vi "G#SubTemplateG3_Create.vi"(0 "reference in":refnum<class "G#SubTemplateG3.lvclass">, 5 "error in (no error)":errorcluster) -> (14 "reference out":refnum<class "G#SubTemplateG3.lvclass">, 19 "error out":errorcluster)   [LabVIEW 2020, in "G#SubTemplateG3.lvclass"]
doc: "Constructor."
uses:
  G#SubTemplateG3.lvclass
  C:/ProjectGSharpDevelopment_2020-3/gsharp/VIPM/Files/vi.lib/addons/_AddQ/G#Object/G#Object.lvclass
  C:/ProjectGSharpDevelopment_2020-3/gsharp/VIPM/Files/vi.lib/addons/_AddQ/G#Templates/G#BaseTemplateG3/G#BaseTemplateG3.lvclass
  G#Object/G#Object.lvclass
  G#BaseTemplateG3/G#BaseTemplateG3.lvclass
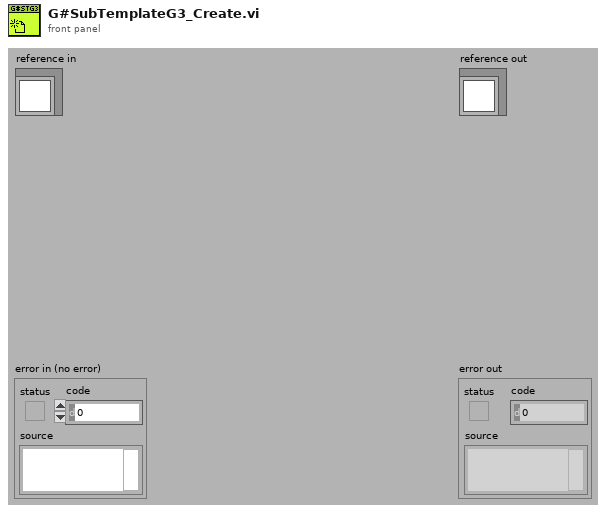
[diagram p1: front panel]
types:
  T1 = typedef "G#SubTemplateG3.lvclass/ObjectAttributes.ctl" = cluster{"Base class":T2}
  T2 = typedef "G#BaseTemplateG3.lvclass/ObjectAttributes.ctl" = cluster{"Numeric":dbl, "String":string, "Boolean":bool}
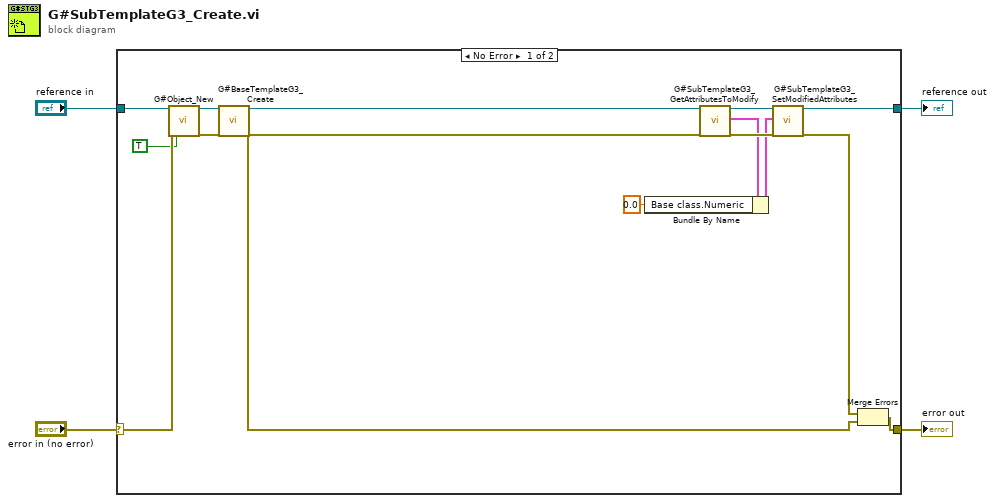
[diagram p0: block diagram]
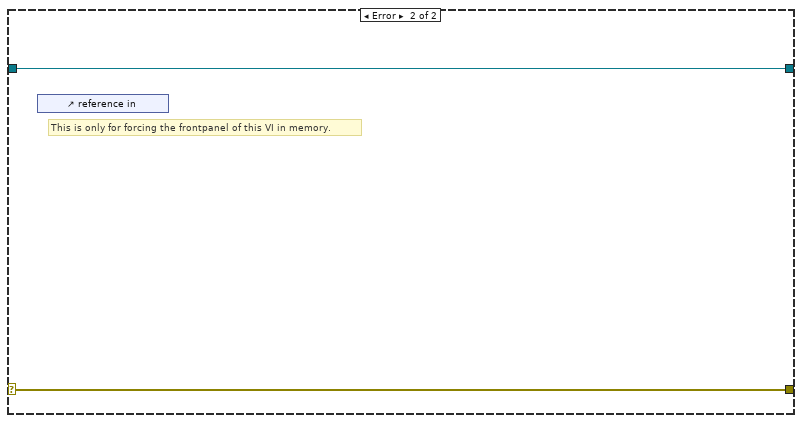
[diagram p2: hidden frame]
diagram:
  n1 = case shown="No Error" "error in (no error)" {
    selector: "error in (no error)" -> [w18 w21]
    tunnel: [w17 w21] -> w3
    tunnel: [w11 w20] -> w1
    tunnel: "reference in" -> [w19 w20]
    frame No Error {
      n2 = call "G#Object_New.vi"("reference in"=w19, "error in (no error)"=w18, "user counter (T)?"=TRUE ("User Counter")) -> ("reference out"=w16:refnum<class "G#SubTemplateG3.lvclass">, "error out"=w15:errorcluster)  [unwired: 14 in, 1 out]
      n3 = call "G#BaseTemplateG3_Create.vi"("reference in"=w16, "error in (no error)"=w15) -> ("reference out"=w12:refnum<class "G#SubTemplateG3.lvclass">, "error out"=w10:errorcluster)  [unwired: 16 in]
      n4 = call "G#SubTemplateG3_GetAttributesToModify.vi"("reference in"=w12, "error in (no error)"=w10) -> ("reference out"=w13:refnum<class "G#SubTemplateG3.lvclass">, "attributes"=w7:T1, "error out"=w9:errorcluster)  [unwired: 13 in, 2 out]
      n5 = Bundle By Name(cluster=w7, "Base class.Numeric"=0.0) -> (w6:T1)
      n6 = call "G#SubTemplateG3_SetModifiedAttributes.vi"("reference in"=w13, "attributes"=w6, "error in (no error)"=w9) -> ("reference out"=w11:refnum<class "G#SubTemplateG3.lvclass">, "error out"=w8:errorcluster)  [unwired: 15 in]
      n7 = Merge Errors(w8, w10) -> (w17:errorcluster)
    }
    frame Error {
      # "This is only for forcing the frontpanel of this VI in memory."
      n8 = control-ref of="reference in"() -> ()  [unwired: 1 out]
    }
  }
  "error out" <- w3
  "reference out" <- w1
